vi "HardwareComm[Poly].vi"   [LabVIEW 2020]
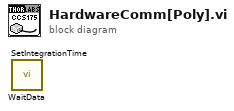
[diagram p0: block diagram]
diagram:
  n1 = call "WaitData.vi"() -> ()  [unwired: 8 in, 4 out]
  n2 = call "SetIntegrationTime.vi"() -> ()  [unwired: 10 in, 2 out]
